vi "picoscopeInitializeSamplingParameters.vi"(11 "PicoscopeV2 in":refnum<class "PicoscopeV2.lvclass">) -> (3 "PicoscopeV2 out":refnum<class "PicoscopeV2.lvclass">)   [LabVIEW 2020, in "PicoscopeV2.lvclass"]
uses:
  PicoscopeV2.lvclass
  PicoscopeV2.lvclass/PicoscopeV2.ctl
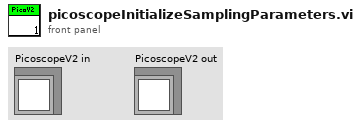
[diagram p1: front panel]
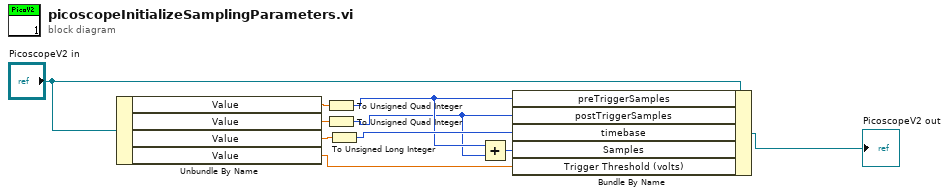
[diagram p0: block diagram]
diagram:
  n1 = Unbundle By Name("PicoscopeV2 in") -> ("Value"=w5:dbl, "Value"=w6:dbl, "Value"=w7:dbl, "Value"=w1:dbl)
  n2 = To Unsigned Quad Integer(1:w5) -> (0:w3:u64)
  n3 = To Unsigned Quad Integer(1:w6) -> (0:w2:u64)
  n4 = To Unsigned Long Integer(number=w7) -> (unsigned 32bit integer=w9:u32)
  n5 = Add(x=w3, y=w2) -> (x+y=w4:u64)
  n6 = Bundle By Name(cluster="PicoscopeV2 in", "preTriggerSamples"=w3, "postTriggerSamples"=w2, "timebase"=w9, "Samples"=w4, "Trigger Threshold (volts)"=w1) -> (→"PicoscopeV2 out":refnum<class "PicoscopeV2.lvclass">)
